vi "Get local language text of controls.vi"(8 "error in (no error)":errorcluster, 11 "Control Label":string="Reference Source") -> (0 "error out":errorcluster, 1 "Values":string[](array[string]), 2 "Control Caption":string, 3 "Control Label":string)   [LabVIEW 2016]
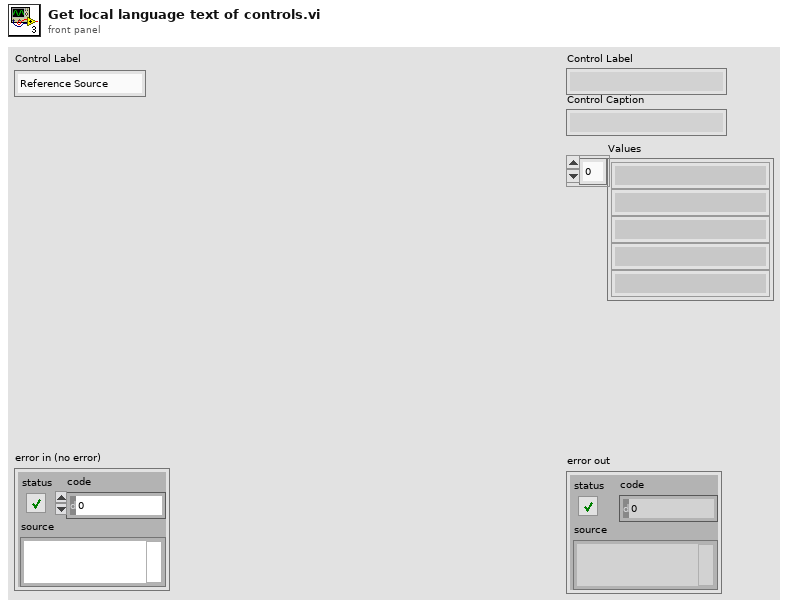
[diagram p1: front panel]
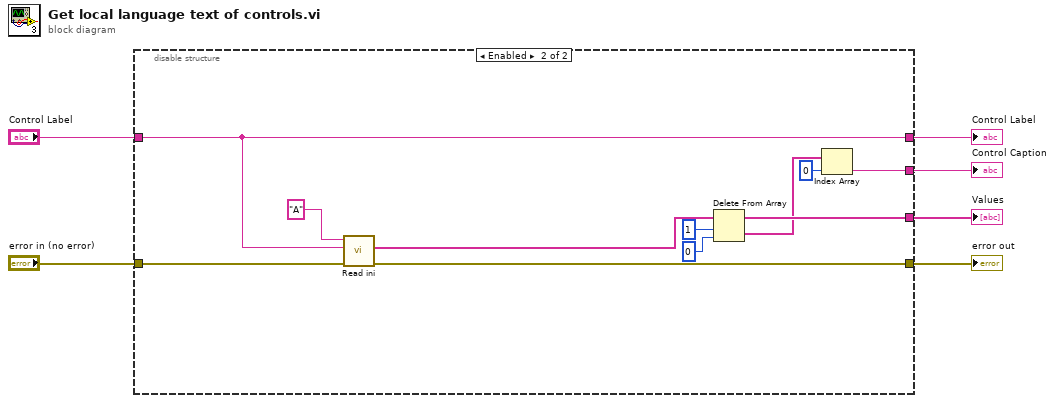
[diagram p0: block diagram]
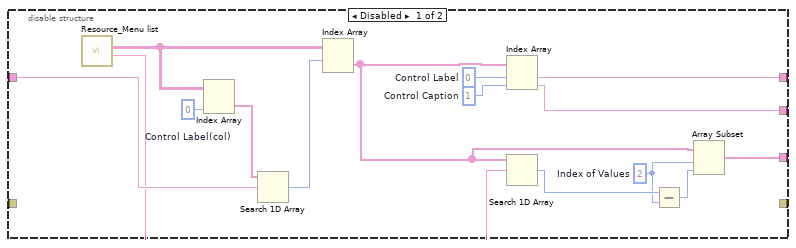
[diagram p2: hidden frame]
diagram:
  n1 = disable-structure shown="Enabled" {
    disable-tunnel: "Control Label" -> [w19 w31]
    disable-tunnel: [w14 w31] -> w5
    disable-tunnel: [w13 w26] -> w4
    disable-tunnel: [w10 w29] -> w3
    disable-tunnel: "error in (no error)" -> [_ w23]
    disable-tunnel: [_ w22] -> w1
    frame Disabled {
      w7 = 2  # Index of Values
      w15 = 1  # Control Caption
      w16 = 0  # Control Label
      w21 = 0  # Control Label(col)
      n2 = call "Resource_Menu list.vi"() -> ("endofvalues"=w12:string, "Resource_Menu list"=w18:string[][])  [unwired: 10 in]
      n3 = Index Array(array=w18, index (col)=w21) -> (element=w20:string[])  [unwired: 1 in]
      n4 = Search 1D Array(1D array=w20, element=w19) -> (index of element=w17:i32)  [unwired: 1 in]
      n5 = Index Array(array=w18, index (row)=w17) -> (element=w9:string[])  [unwired: 1 in]
      n6 = Index Array(array=w9, index #1=w16, index #2=w15) -> (element #1=w14:string, element #2=w13:string)
      n7 = Search 1D Array(1D array=w9, element=w12) -> (index of element=w11:i32)  [unwired: 1 in]
      n8 = Subtract(x=w11, y=w7) -> (x-y=w8:i32)
      n9 = Array Subset(array=w9, index=w7, length=w8) -> (w10:string[])
    }
    frame Enabled {
      n10 = call "Read ini.vi"("error in (no error)"=w23, "key"=w31, "section"="A") -> ("error out"=w22:errorcluster, "Value"=w30:string[])  [unwired: 7 in]
      n11 = Delete From Array(array=w30, length=1, index=0) -> (deleted portion=w25:string[], array with subset deleted=w29:string[])
      n12 = Index Array(array=w25, index=0) -> (element=w26:string)
    }
  }
  "Control Label" <- w5
  "Control Caption" <- w4
  "Values" <- w3
  "error out" <- w1
